vi "ConvertVIFunctionToString.vi"(11 "Function":enum16{"Voltage", "Current"}(ring)) -> (3 "Function (v or i)":string)   [LabVIEW 2012, in "Keithley-2602.lvlib"]
uses:
  Keithley-2602.lvlib
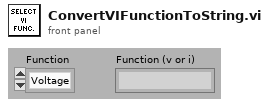
[diagram p1: front panel]
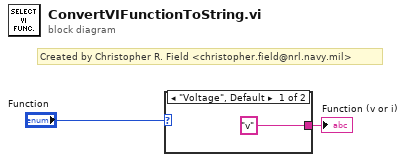
[diagram p0: block diagram]
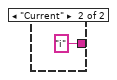
[diagram p2: hidden frame]
diagram:
  # "Created by Christopher R. Field <christopher.field@nrl.navy.mil>"
  n1 = case shown="\"Voltage\", Default" "Function" {
    tunnel: ["v" "i"] -> w2
    frame "Voltage", Default {
    }
    frame "Current" {
    }
  }
  "Function (v or i)" <- w2
